vi "ScissorLift.vi"(1 "Down":bool, 2 "Up":bool) -> ()   [LabVIEW 2014]
panel:
  out "Bottom":bool
  out "Top":bool
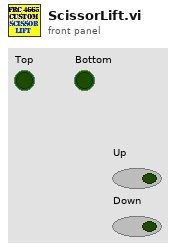
[diagram p1: front panel]
types:
  T1 = typedef "WPI_DigitalInputDevRef.ctl" = cluster{"DevStatus":errorcluster, "DIO Channel":T2, "Controller":T3}
  T2 = typedef "FPGA_DIOChannel.ctl" = enum8{"DIO 0", "DIO 1", "DIO 2", "DIO 3", "DIO 4", "DIO 5", "DIO 6", "DIO 7", "DIO 8", "DIO 9", "DIO MXP 0", "DIO MXP 1", "DIO MXP 2", "DIO MXP 3", "DIO MXP 4", "DIO MXP 5", "DIO MXP 6", "DIO MXP 7", "DIO MXP 8", "DIO MXP 9", "DIO MXP 10", "DIO MXP 11", "DIO MXP 12", "DIO MXP 13", "DIO MXP 14", "DIO MXP 15", "Invalid"}
  T3 = typedef "FPGA_TypedefDigitalModule.ctl" = enum16{"Controller 1"}
  T4 = typedef "WPI_MotorControlDeviceRef.ctl" = cluster{"DeviceStatus":errorcluster, "Type":T5, "PWM":cluster{"Controller":T3, "PWM Channel":T6, "DeadBand":T7}, "CAN":cluster{"Device Number":u8, "Control Mode":T8, "Semaphore":T9, "Max Vout":dbl, "TalonSRX Control Mode":T10}, "Invert":bool, "TransformRef":T11, "InvTransformRef":T11}
  T5 = typedef "WPI_MotorControlType.ctl" = enum16{"PWM", "CAN", "CANTalonSRX"}
  T6 = typedef "FPGA_DIOPWMChannel.ctl" = enum8{"PWM 0", "PWM 1", "PWM 2", "PWM 3", "PWM 4", "PWM 5", "PWM 6", "PWM 7", "PWM 8", "PWM 9", "PWM MXP 0", "PWM MXP 1", "PWM MXP 2", "PWM MXP 3", "PWM MXP 4", "PWM MXP 5", "PWM MXP 6", "PWM MXP 7", "PWM MXP 8", "PWM MXP 9", "Invalid"}
  T7 = typedef "WPI_PWMDeadband.ctl" = cluster{"Name":string, "maxPositivePwm":i32, "minPositivePwm":i32, "centerPwm":i32, "maxNegativePwm":i32, "minNegativePwm":i32, "angularRange":u16}
  T8 = typedef "WPI_CANJaguar_ControlMode.ctl" = enum8{"Percent VBus", "Current", "Speed", "Position", "Voltage"}
  T9 = typedef "Semaphore RefNum" = refnum<k1>
  T10 = typedef "WPI_CANTalonSRX_APIControlMode.ctl" = enum8{"Percent VBus", "Speed", "Position", "Slave", "Unchanged / Invalid"}
  T11 = typedef "WPI_PWMTransform_ConPane.ctl" = refnum<vi>
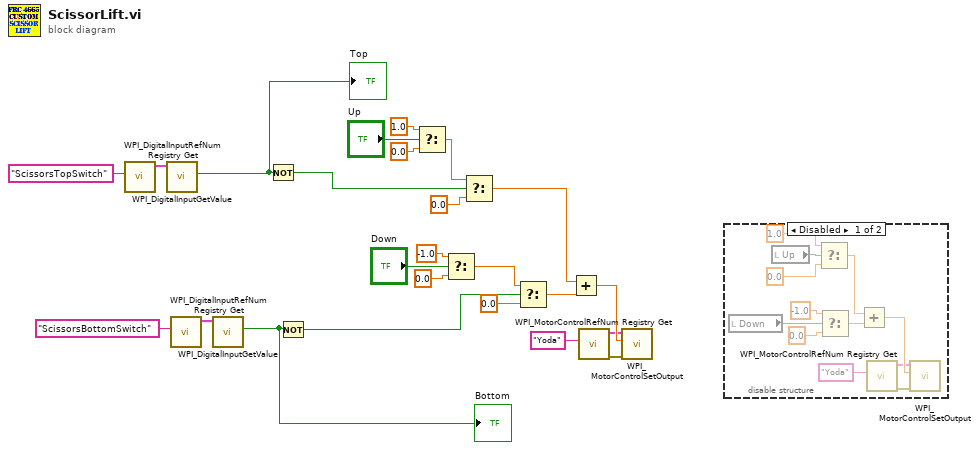
[diagram p0: block diagram]
diagram:
  n1 = call <vilib>:"WPI_DigitalInputRefNum Registry Get.vi"("refnum name"="ScissorsTopSwitch") -> ("DigitalInputDevRef"=w13:T1)  [unwired: 9 in, 1 out]
  n2 = call <vilib>:"WPI_DigitalInputGetValue.vi"("DigitalInputDevRef"=w13) -> ("Value"=w23:bool)  [unwired: 8 in, 2 out]
  "Top" <- w23
  n3 = call <vilib>:"WPI_DigitalInputRefNum Registry Get.vi"("refnum name"="ScissorsBottomSwitch") -> ("DigitalInputDevRef"=w19:T1)  [unwired: 9 in, 1 out]
  n4 = call <vilib>:"WPI_DigitalInputGetValue.vi"("DigitalInputDevRef"=w19) -> ("Value"=w24:bool)  [unwired: 8 in, 2 out]
  "Bottom" <- w24
  n5 = Not(x=w23) -> (.not. x?=w21:bool)
  n6 = Not(x=w24) -> (.not. x?=w22:bool)
  n7 = Select(t=1.0, s="Up", f=0.0) -> (s? t:f=w12:dbl)
  n8 = Select(t=-1.0, s="Down", f=0.0) -> (s? t:f=w17:dbl)
  n9 = Select(t=w12, s=w21, f=0.0) -> (s? t:f=w14:dbl)
  n10 = Select(t=w17, s=w22, f=0.0) -> (s? t:f=w16:dbl)
  n11 = Add(x=w14, y=w16) -> (x+y=w8:dbl)
  n12 = call <vilib>:"WPI_MotorControlRefNum Registry Get.vi"("refnum name"="Yoda") -> ("error out"=w1:errorcluster, "MotorControlDevRef"=w2:T4)  [unwired: 9 in]
  n13 = call <vilib>:"WPI_MotorControlSetOutput.vi"("error in (no error)"=w1, "Output"=w8, "MotorControlDevRef"=w2) -> ()  [unwired: 6 in, 3 out]
  n14 = disable-structure shown="Disabled" {
    frame Disabled {
      n15 = local read "Down"() -> (w36:bool)
      n16 = local read "Up"() -> (w35:bool)
      n17 = Select(t=1.0, s=w35, f=0.0) -> (s? t:f=w33:dbl)
      n18 = Select(t=-1.0, s=w36, f=0.0) -> (s? t:f=w34:dbl)
      n19 = Add(x=w33, y=w34) -> (x+y=w32:dbl)
      n20 = call <vilib>:"WPI_MotorControlRefNum Registry Get.vi"("refnum name"="Yoda") -> ("error out"=w25:errorcluster, "MotorControlDevRef"=w26:T4)  [unwired: 9 in]
      n21 = call <vilib>:"WPI_MotorControlSetOutput.vi"("error in (no error)"=w25, "Output"=w32, "MotorControlDevRef"=w26) -> ()  [unwired: 6 in, 3 out]
    }
    frame Enabled {
    }
  }
